vi "Test_LogIfError_WarningFlagged_WarningLogged.vi"(8 "error in (no error)":errorcluster, 11 "TestCase in":refnum<class "TestComposedLog.lvclass">) -> (0 "error out":errorcluster, 3 "TestCase out":refnum<class "TestComposedLog.lvclass">)   [LabVIEW 2017, in "TestComposedLog.lvclass"]
uses:
  TestComposedLog.lvclass
  Source/Composed Log/Types/Log Level.ctl
  Source/Composed Log/LoggerReference/LoggerReference.lvclass/LoggerReference.ctl
  Source/LVQueue Sink/LVQueue Sink.lvclass/LVQueue Sink.ctl
  30b30c6e-1cbf-4399-a934-057b2bffe360.vi
  30b30c6e-1cbf-4399-a934-057b2bffe360.vi/956d482e-ee10-4565-9360-1d129b9619a1.vi
  Source/Composed Log/LoggerReference/Return Aggregate Queues.vi
  Source/Composed Log/LoggerReference/Add Aggregate Log.vi
  30b30c6e-1cbf-4399-a934-057b2bffe360.vi/956d482e-ee10-4565-9360-1d129b9619a1.vi/9a528c4c-d8d7-4db3-a957-385c7eca20b3.vi
  Source/Composed Log/LoggerReference/Send Add Sink.vi
  Source/LVQueue Sink/LVQueue Sink.lvclass
  C:/CS/Internal/LabVIEW/Logger/Source/Composed Log/Log Sink/Log Sink.lvclass
  Source/Composed Log/Application Logger/Launch Worker Loop.vi
  Source/Composed Log/LoggerReference/Initialize Logger Instance.vi
  Source/Composed Log/Singleton Event Log/Logger Queue FGV.vi
  Source/Composed Log/IErrorFormat/IErrorFormat.lvclass
  Source/Composed Log/LoggerReference/LoggerReference.lvclass
  Source/Composed Log/Log Sink/Log Sink.lvclass
  <vilib>/addons/_JKI Toolkits/VI Tester/TestCase.llb/TestCase.lvclass
  Source/Composed Log/Singleton Event Log/Singleton Event Log.lvlib
  Source/Composed Log/Composed Log.lvlib
  C:/Program Files (x86)/National Instruments/LabVIEW 2017/vi.lib/addons/_JKI Toolkits/VI Tester/TestCase.llb/TestCase.lvclass
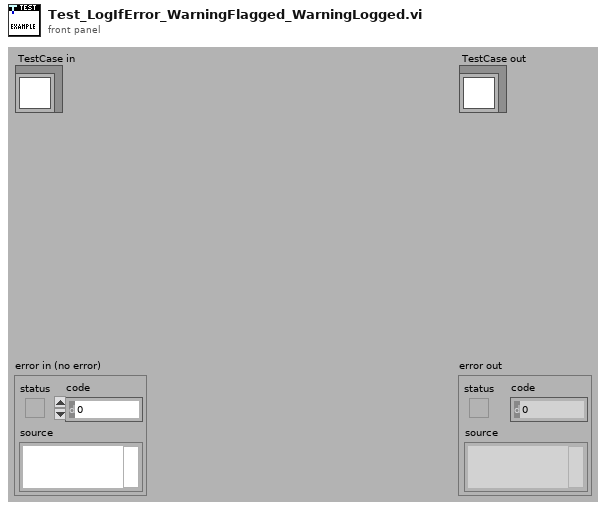
[diagram p1: front panel]
types:
  T1 = typedef "Composed Log.lvlib/Log Level.ctl" = enum16{"Debug", "Info", "Warning", "Error", "Critical"}
  T2 = typedef "Composed Log.lvlib/Log Packet.ctl" = cluster{"Data To Log":string, "Source":string, "Event Level":T1, "Event Time":timestamp}
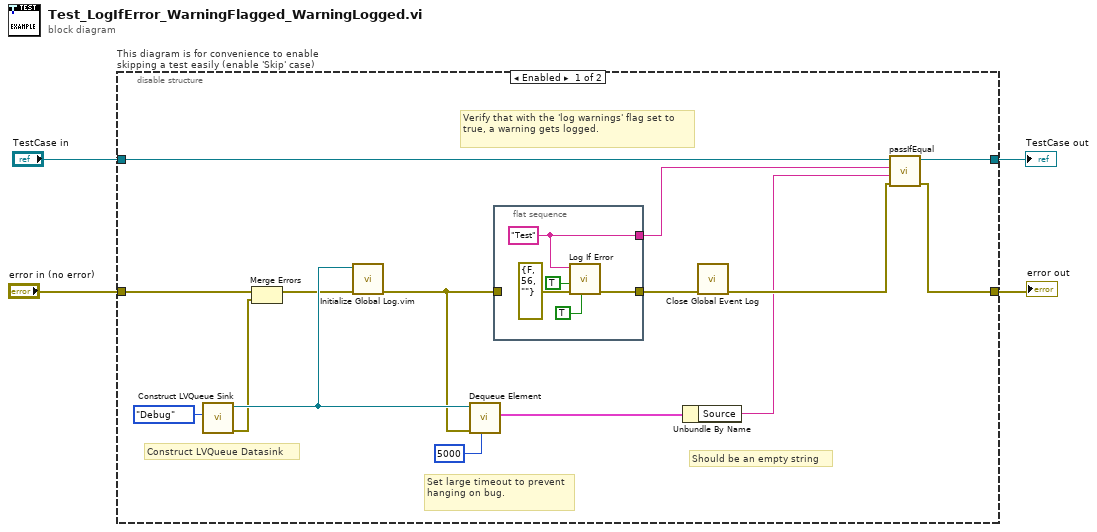
[diagram p0: block diagram]
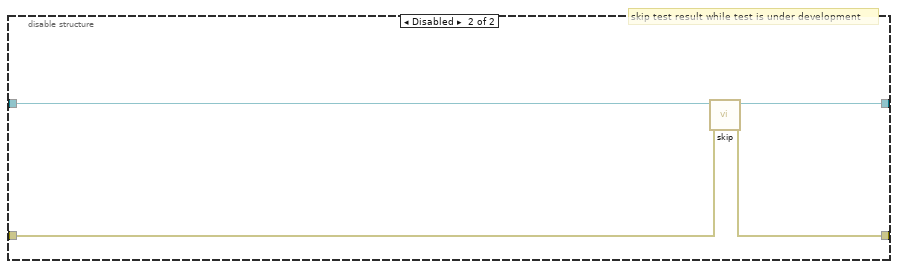
[diagram p2: hidden frame]
diagram:
  n1 = disable-structure "This diagram is for convenience to enable skipping a test easily (enable 'Skip' case)" shown="Enabled" {
    disable-tunnel: "TestCase in" -> [w8 w28]
    disable-tunnel: [w7 w26] -> w1
    disable-tunnel: [w9 w27] -> w3
    disable-tunnel: "error in (no error)" -> [w19 w25]
    frame Enabled {
      # "Should be an empty string"
      # "Construct LVQueue Datasink"
      # "Set large timeout to prevent hanging on bug."
      # "Verify that with the 'log warnings' flag set to true, a warning gets logged."
      n2 = call "Construct LVQueue Sink.vi"("LogLevel"=Log_Level."Debug") -> ("error out"=w13:errorcluster, "LVQueue Sink out"=w17:refnum<class "LVQueue Sink.lvclass">)  [unwired: 9 in]
      n3 = Merge Errors(w19, w13) -> (w14:errorcluster)
      n4 = call "Initialize Global Log.vim"("error in (no error)"=w14, "Log Sink(s)"=w17) -> ("error out"=w12:errorcluster)  [unwired: 8 in, 1 out]
      n5 = call "Dequeue Element.vi"("timeout in ms (-1)"=5000, "error in (no error)"=w12, "LVQueue Sink in"=w17) -> ("Log Packet"=w15:T2)  [unwired: 5 in, 3 out]
      n6 = flat-sequence {
        tunnel: w12 -> [_]
        tunnel: [w21] -> w11
        tunnel: [w22] -> w5
        frame #0 {
          w22 = "Test" ("SourceID")
          n7 = call "Log If Error.vi"("Include Warnings(F)"=TRUE, "Error In"=errorcluster {"status"=FALSE, "code"=56, "source"=""}, "Clear After Logging?(F)"=TRUE, "SourceID"=w22) -> ("error out"=w21:errorcluster)  [unwired: 7 in]
        }
      }
      n8 = Unbundle By Name(w15) -> ("Source"=w6:string)
      n9 = call "Close Global Event Log.vi"("error in (no error)"=w11) -> ("error out"=w10:errorcluster)  [unwired: 10 in]
      n10 = call-dynamic "passIfEqual.vi"("error in (no error)"=w10, "y"=w6, "x"=w5, "TestCase in"=w8) -> ("error out"=w9:errorcluster, "TestCase out"=w7:refnum<class "TestComposedLog.lvclass">)  [unwired: 6 in]
    }
    frame Disabled {
      # "skip test result while test is under development"
      n11 = call <vilib>:"skip.vi"("error in (no error)"=w25, "TestCase in"=w28) -> ("error out"=w27:errorcluster, "TestCase out"=w26:refnum<class "TestComposedLog.lvclass">)  [unwired: 8 in]
    }
  }
  "error out" <- w3
  "TestCase out" <- w1
